vi "VPA QC Graph Size.vi"(10 "State Cluster":T1) -> (2 "State Cluster Out":T1)   [LabVIEW 2013]
uses:
  Controls/VPA QC State Data Cluster.ctl
  Controls/VPA QC General Cluster.ctl
  Controls/VPA QC State Enum.ctl
  Controls/VPA QC Bool Cluster.ctl
panel:
  in  "Export Graph":bool
  in  "Exit":bool
  in  "Data to Display":T5(ring)
  out "Waveform Graph":waveform(dbl)[](graph) caption="Pressure Test"
  # "Assembly Checklist"
  # "Assembly Checklist"
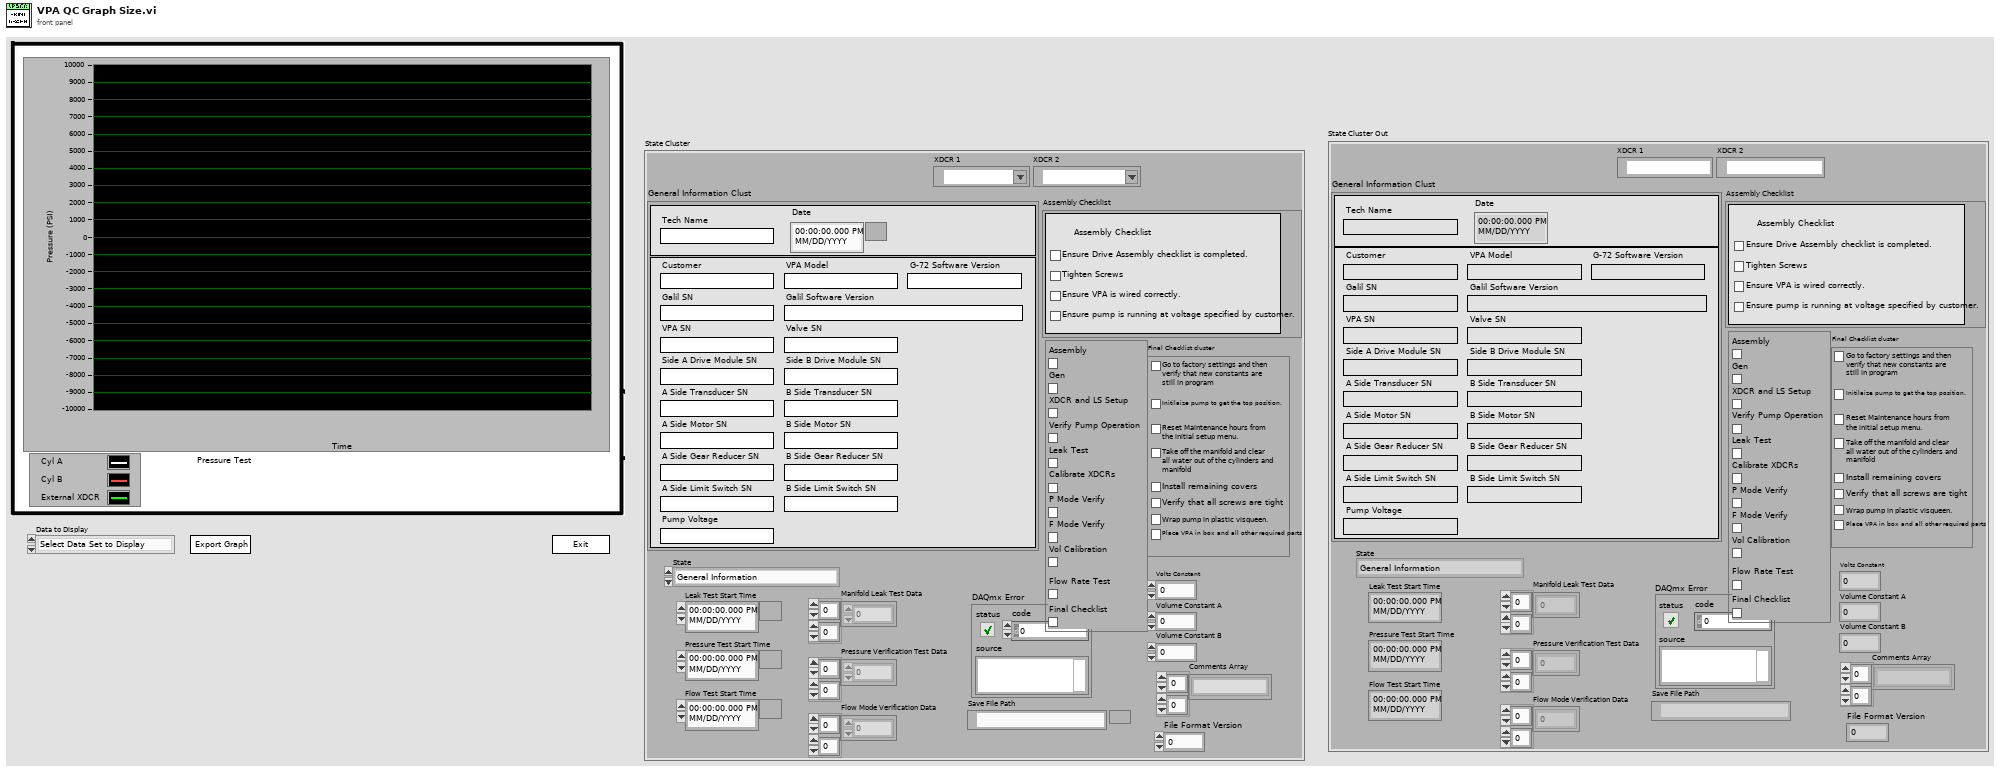
[diagram p1: front panel]
types:
  T1 = typedef "VPA QC State Data Cluster.ctl" = cluster{"XDCR 1":tag, "XDCR 2":tag, "General Information Clust":T2, "Assembly Checklist":cluster{"Ensure Drive Assembly checklist is completed.":bool, "Tighten Screws":bool, "Ensure VPA is wired correctly.":bool, "Ensure pump is running at voltage specified by customer.":bool}, "State":T3, "Manifold Leak Test Data":dbl[][], "Pressure Verification Test Data":dbl[][], "Flow Mode Verification Data":dbl[][], "DAQmx Error":errorcluster, "Bool Cluster":T4, "Leak Test Start Time":timestamp, "Pressure Test Start Time":timestamp, "Flow Test Start Time":timestamp, "Final Checklist cluster":cluster{"Check Fact Rest":bool, "Initialize Pump":bool, "Maintenance Hours":bool, "Clean Water Out":bool, "Covers":bool, "Screws":bool, "Wrap":bool, "Box":bool}, "Volts Constant":dbl, "Volume Constant A":dbl, "Volume Constant B":dbl, "Save File Path":path, "Comments Array":string[][], "File Format Version":u16}
  T2 = typedef "VPA QC General Cluster.ctl" = cluster{"Tech Name":string, "Date":timestamp, "Customer":string, "VPA Model":string, "G-72 Software Version":string, "Galil SN":string, "Galil Software Version":string, "VPA SN":string, "Valve SN":string, "Side A Drive Module SN":string, "Side B Drive Module SN":string, "A Side Transducer SN":string, "B Side Transducer SN":string, "A Side Motor SN":string, "B Side Motor SN":string, "A Side Gear Reducer SN":string, "B Side Gear Reducer SN":string, "A Side Limit Switch SN":string, "B Side Limit Switch SN":string, "Pump Voltage":string}
  T3 = typedef "VPA QC State Enum.ctl" = enum16{"General Information", "XDCR and LS Check", "Check Pump Function", "Manifold/Cylinder Leak Test", "Exit"}
  T4 = typedef "VPA QC Bool Cluster.ctl" = cluster{"Assembly":bool, "Gen":bool, "XDCR and LS Setup":bool, "Verify Pump Operation":bool, "Leak Test":bool, "Calibrate XDCRs":bool, "P Mode Verify":bool, "F Mode Verify":bool, "Vol Calibration":bool, "Flow Rate Test":bool, "Final Checklist":bool}
  T5 = enum16{"Select Data Set to Display", "Leak Test", "Pressure Test", "Flow Test"}
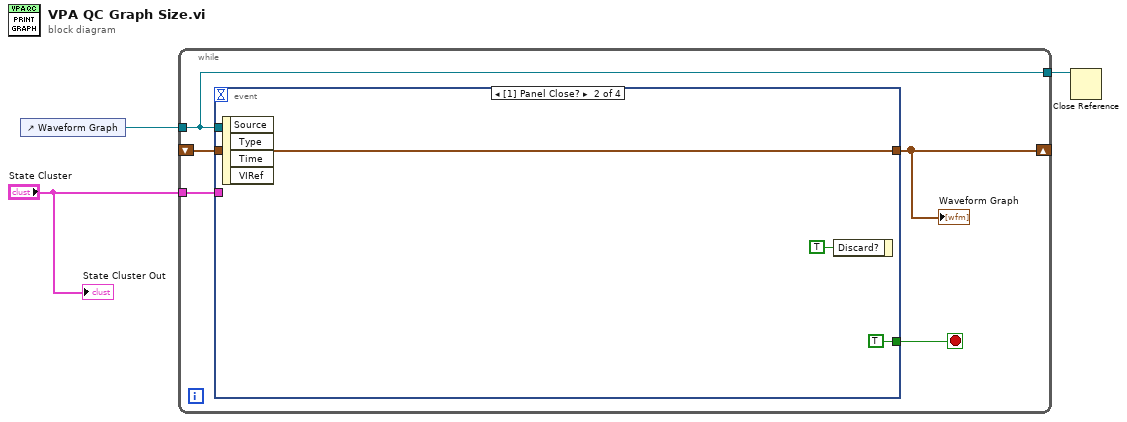
[diagram p0: block diagram]
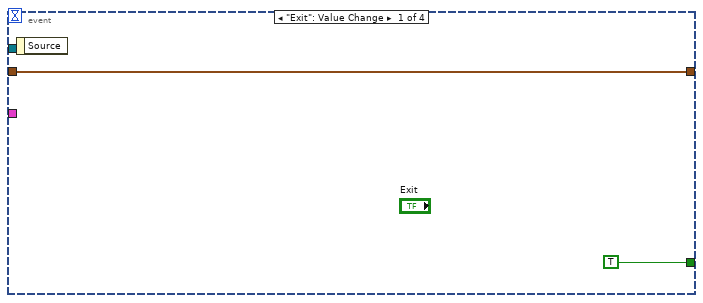
[diagram p2: hidden frame]
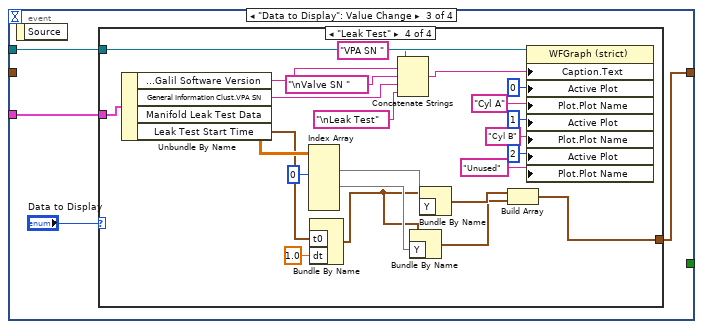
[diagram p3: hidden frame]
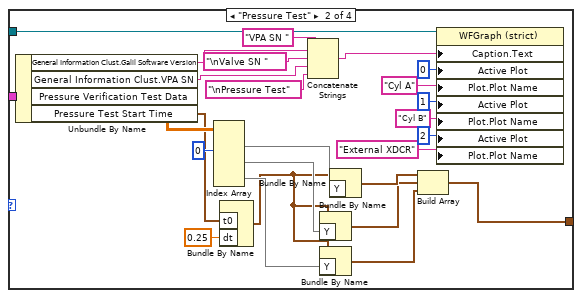
[diagram p5: hidden frame]
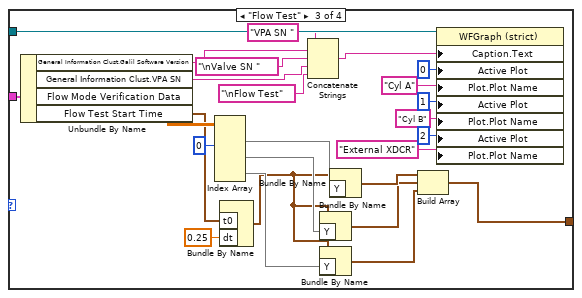
[diagram p6: hidden frame]
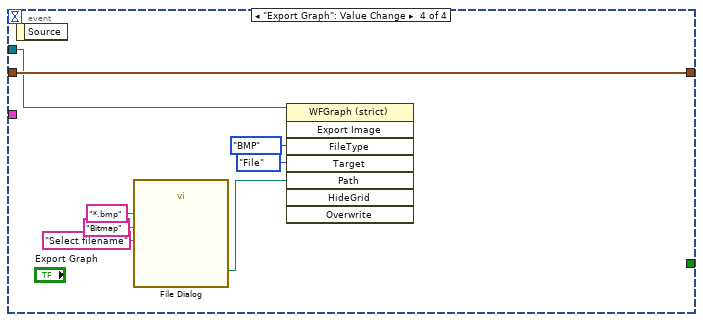
[diagram p7: hidden frame]
diagram:
  n1 = control-ref of="Waveform Graph"() -> (w2:refnum<vi>)
  n2 = while {
    tunnel: "State Cluster" -> [w7]
    shift-right: [w6] -> _
    shift-left: _ -> [w5]
    tunnel: w2 -> [w4]
    tunnel: [w4] -> w1
    stop <- w8 stop-if-true
    n3 = event shown="[1] Panel Close?" {
      selector: _ -> [_ _ _ _]
      dyn-events: _ -> [_ _ _ _]
      timeout: _ -> [_ _ _ _]
      tunnel: [TRUE TRUE _ _] -> w8
      tunnel: w7 -> [_ _ w17 _]
      tunnel: [w9 w13 w16 w101] -> w6
      tunnel: w5 -> [w9 w13 _ w101]
      tunnel: w4 -> [_ _ w15 w100]
      event "Exit": Value Change {
        n4 = event-data() -> ()  [unwired: 1 in, 1 out]
      }
      event Panel Close? {
        n5 = event-data() -> ()  [unwired: 1 in, 4 out]
        n6 = event-data("Discard?"=TRUE) -> ()  [unwired: 1 in, 1 out]
      }
      event "Data to Display": Value Change {
        n7 = event-data() -> ()  [unwired: 1 in, 1 out]
        n8 = case shown="\"Leak Test\"" "Data to Display" {
          tunnel: w17 -> [_ w43 w69 w93]
          tunnel: [_ w37 w63 w87] -> w16
          tunnel: w15 -> [_ w36 w62 w86]
          frame "Select Data Set to Display" {
          }
          frame "Pressure Test" {
            n9 = Unbundle By Name(w43) -> ("General Information Clust.Galil Software Version"=w22:string, "General Information Clust.VPA SN"=w18:string, "Pressure Verification Test Data"=w42:dbl[][], "Pressure Test Start Time"=w26:timestamp)
            n10 = Index Array(array=w42, index (col) #1=0 ("disabled index (col)")) -> (element #1=w41:dbl[], element #2=w40:dbl[], element #3=w31:dbl[])  [unwired: 5 in]
            n11 = Bundle By Name("t0"=w26, "dt"=0.25) -> (w24:waveform(dbl))  [unwired: 1 in]
            n12 = Concatenate Strings("VPA SN " ("string"), w22, "\nValve SN " ("string"), w18, "\nPressure Test" ("string")) -> (w21:string)
            n13 = Bundle By Name(cluster=w24, "Y"=w40) -> (w38:waveform(dbl))
            n14 = Bundle By Name(cluster=w24, "Y"=w31) -> (w30:waveform(dbl))
            n15 = Bundle By Name(cluster=w24, "Y"=w41) -> (w39:waveform(dbl))
            n16 = Build Array(w39, w38, w30) -> (w37:waveform(dbl)[])
            n17 = property class="WFGraph (strict)"(reference=w36, "Caption.Text"=w21, "Active Plot"=u32 0, "Plot.Plot Name"="Cyl A", "Active Plot"=u32 1, "Plot.Plot Name"="Cyl B", "Active Plot"=u32 2, "Plot.Plot Name"="External XDCR") -> ()  [unwired: 1 in, 2 out]
          }
          frame "Flow Test" {
            n18 = Unbundle By Name(w69) -> ("General Information Clust.Galil Software Version"=w48:string, "General Information Clust.VPA SN"=w45:string, "Flow Mode Verification Data"=w68:dbl[][], "Flow Test Start Time"=w52:timestamp)
            n19 = Index Array(array=w68, index (col) #1=0 ("disabled index (col)")) -> (element #1=w67:dbl[], element #2=w66:dbl[], element #3=w57:dbl[])  [unwired: 5 in]
            n20 = Bundle By Name("t0"=w52, "dt"=0.25) -> (w50:waveform(dbl))  [unwired: 1 in]
            n21 = Concatenate Strings("VPA SN " ("string"), w48, "\nValve SN " ("string"), w45, "\nFlow Test" ("string")) -> (w47:string)
            n22 = Bundle By Name(cluster=w50, "Y"=w66) -> (w64:waveform(dbl))
            n23 = Bundle By Name(cluster=w50, "Y"=w57) -> (w56:waveform(dbl))
            n24 = Bundle By Name(cluster=w50, "Y"=w67) -> (w65:waveform(dbl))
            n25 = Build Array(w65, w64, w56) -> (w63:waveform(dbl)[])
            n26 = property class="WFGraph (strict)"(reference=w62, "Caption.Text"=w47, "Active Plot"=u32 0, "Plot.Plot Name"="Cyl A", "Active Plot"=u32 1, "Plot.Plot Name"="Cyl B", "Active Plot"=u32 2, "Plot.Plot Name"="External XDCR") -> ()  [unwired: 1 in, 2 out]
          }
          frame "Leak Test" {
            n27 = Unbundle By Name(w93) -> ("General Information Clust.Galil Software Version"=w74:string, "General Information Clust.VPA SN"=w71:string, "Manifold Leak Test Data"=w92:dbl[][], "Leak Test Start Time"=w78:timestamp)
            n28 = Index Array(array=w92, index (col) #1=0 ("disabled index (col)")) -> (element #1=w91:dbl[], element #2=w90:dbl[])  [unwired: 5 in, 1 out]
            n29 = Bundle By Name("t0"=w78, "dt"=1.0) -> (w76:waveform(dbl))  [unwired: 1 in]
            n30 = Concatenate Strings("VPA SN " ("string"), w74, "\nValve SN " ("string"), w71, "\nLeak Test" ("string")) -> (w73:string)
            n31 = Bundle By Name(cluster=w76, "Y"=w90) -> (w88:waveform(dbl))
            n32 = Bundle By Name(cluster=w76, "Y"=w91) -> (w89:waveform(dbl))
            n33 = Build Array(w89, w88) -> (w87:waveform(dbl)[])
            n34 = property class="WFGraph (strict)"(reference=w86, "Caption.Text"=w73, "Active Plot"=u32 0, "Plot.Plot Name"="Cyl A", "Active Plot"=u32 1, "Plot.Plot Name"="Cyl B", "Active Plot"=u32 2, "Plot.Plot Name"="Unused") -> ()  [unwired: 1 in, 2 out]
          }
        }
      }
      event "Export Graph": Value Change {
        n35 = event-data() -> ()  [unwired: 1 in, 1 out]
        n36 = call "File Dialog"("prompt"="Select filename", "pattern (all files)"="*.bmp", "pattern label"="Bitmap") -> ("selected path"=w97:path)  [unwired: 9 in, 3 out]
        n37 = invoke class="WFGraph (strict)" method="Export Image"(reference=w100, "FileType"=enum32{"BMP", "EPS", "EMF", "PICT"}."BMP" ("File Type"), "Target"=enum32{"File", "Clipboard"}."File", "Path"=w97) -> ()  [unwired: 4 in, 8 out]
      }
    }
    "Waveform Graph" <- w6
  }
  n38 = Close Reference(reference=w1) -> ()  [unwired: 1 in, 1 out]
  "State Cluster Out" <- "State Cluster"
